vi "CtrlTreeReload.vi"(8 "error in (no error)":errorcluster, 11 "TreeControl in":refnum<vi>) -> (0 "error out":errorcluster, 3 "TreeControl out":refnum<vi>)   [LabVIEW 2021]
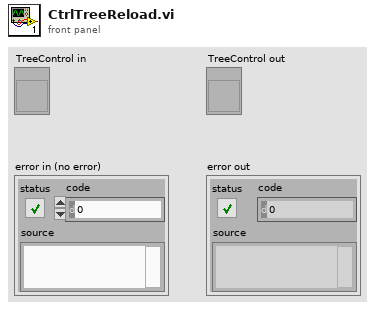
[diagram p1: front panel]
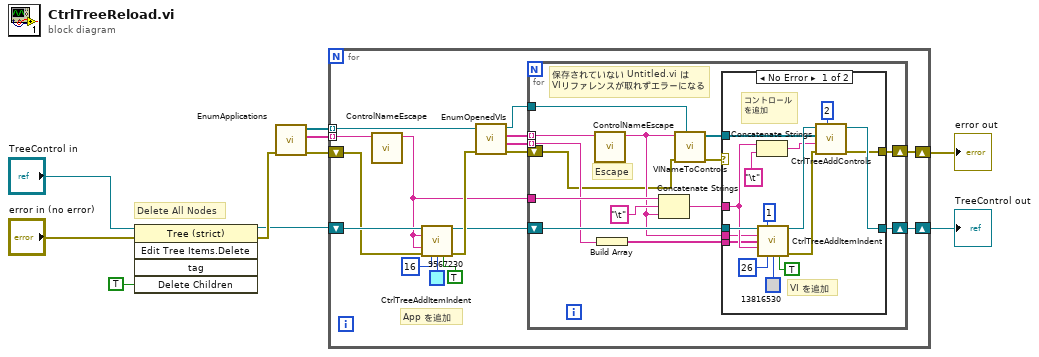
[diagram p0: block diagram]
diagram:
  # "Delete All Nodes"
  n1 = invoke class="Tree (strict)" method="Edit Tree Items.Delete"(reference="TreeControl in", error in="error in (no error)", "Delete Children"=TRUE ("Delete Children?")) -> (reference out=w7:refnum<vi>, error out=w8:errorcluster)  [unwired: 2 in, 3 out]
  n2 = call "EnumApplications.vi"("error in (no error)"=w8) -> ("error out"=w5:errorcluster, "Application Names"=w9:string[], "Application References"=w4:refnum<vi>[])  [unwired: 8 in]
  n3 = for {
    tunnel: w4 -> [w15] mode=indexing
    shift-right: [w19] -> w1
    shift-left: w5 -> [w17]
    tunnel: w9 -> [w18] mode=indexing
    shift-right: [w16] -> w2
    shift-left: w7 -> [w26]
    # "App を追加"
    n4 = call "ControlNameEscape.vi"("label"=w18) -> ("escaped string"=w11:string)  [unwired: 10 in]
    n5 = call "CtrlTreeAddItemIndent.vi"("TreeControl in"=w26, "Left Cell String"=w11, "Tag"=w11, "error in (no error)"=w17, "Symbol Index"=16, "Background Color"=u32 9567230, "Bold Font"=TRUE) -> ("TreeControl out"=w22:refnum<vi>, "error out"=w25:errorcluster)  [unwired: 6 in, 1 out]
    n6 = call "EnumOpenedVIs.vi"("error in (no error)"=w25, "Application in"=w15) -> ("error out"=w20:errorcluster, "Positions"=w13:string[], "VI Tags"=w14:string[], "Application out"=w12:refnum<vi>)  [unwired: 6 in]
    n7 = for {
      tunnel: w14 -> [w31] mode=indexing
      tunnel: w11 -> [w39]
      shift-right: [w27] -> w19
      shift-left: w20 -> [w29]
      shift-right: [w35] -> w16
      shift-left: w22 -> [w40]
      tunnel: w12 -> [w36]
      tunnel: w13 -> [w33] mode=indexing
      # "Escape"
      # "保存されていない Untitled.vi は\nVIリファレンスが取れずエラーになる"
      n8 = call "ControlNameEscape.vi"("label"=w31) -> ("escaped string"=w30:string)  [unwired: 10 in]
      n9 = Build Array(w33) -> (w32:string[])
      n10 = Concatenate Strings(w39, "\t" ("string"), w30) -> (w34:string)
      n11 = call "VINameToControls.vi"("application reference (local)"=w36, "error in (no error)"=w29, "vi"=w30) -> ("error out"=w28:errorcluster, "FlattenControls[]"=w37:refnum<vi>[])  [unwired: 6 in, 1 out]
      n12 = case shown="No Error" w28 {
        tunnel: w40 -> [w56 w57]
        tunnel: w37 -> [w50 _]
        tunnel: [w49 w57] -> w35
        tunnel: w34 -> [w46 _]
        tunnel: w32 -> [w44 _]
        tunnel: w30 -> [w43 _]
        tunnel: [w42 _] -> w27
        frame No Error {
          # "VI を追加"
          # "コントロール\nを追加"
          n13 = Concatenate Strings(w46, "\t" ("string")) -> (w45:string)
          n14 = call "CtrlTreeAddItemIndent.vi"("TreeControl in"=w56, "Indentation"=1, "Left Cell String"=w43, "Child Text"=w44, "Tag"=w46, "Symbol Index"=26, "Background Color"=u32 13816530, "Bold Font"=TRUE) -> ("TreeControl out"=w51:refnum<vi>, "error out"=w41:errorcluster)  [unwired: 5 in, 1 out]
          n15 = call "CtrlTreeAddControls.vi"("Indentation"=2, "error in (no error)"=w41, "Path"=w45, "Controls[]"=w50, "TreeControl in"=w51) -> ("error out"=w42:errorcluster, "TreeControl out"=w49:refnum<vi>)  [unwired: 5 in]
        }
        frame Error {
        }
      }
    }
  }
  "error out" <- w1
  "TreeControl out" <- w2
